vi "Log_Show.vi"() -> (1 "Log Out":string)   [LabVIEW 2020]
panel:
  out "Itterations":i32
  out "ticks":u32
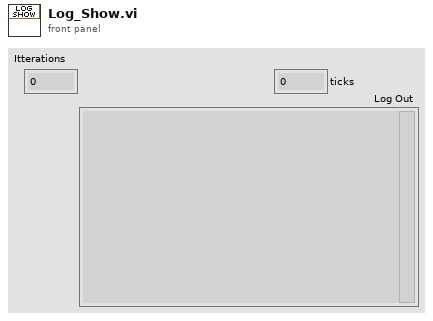
[diagram p1: front panel]
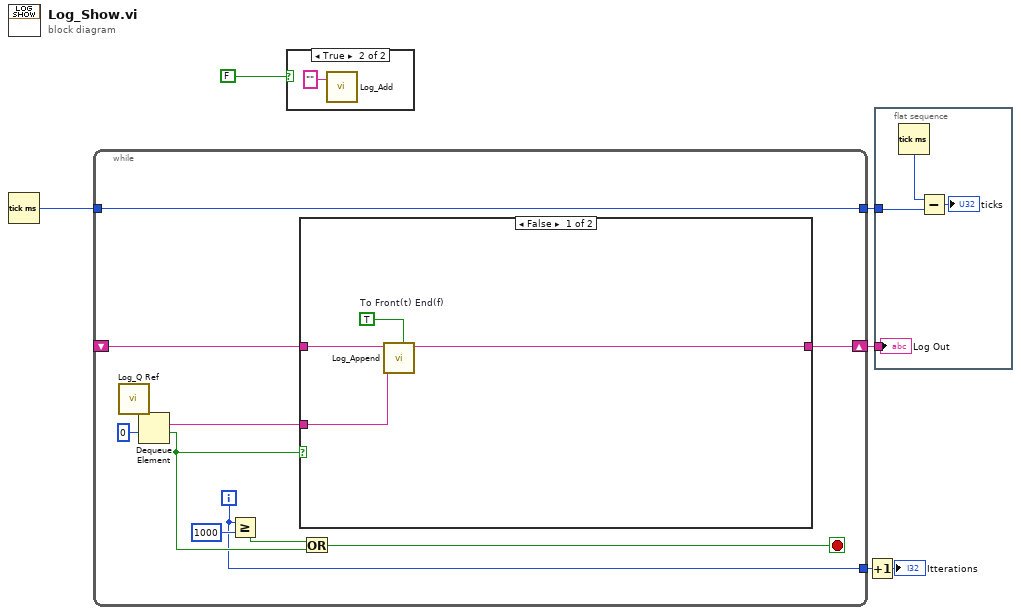
[diagram p0: block diagram]
diagram:
  n1 = Tick Count (ms)() -> (millisecond timer value=w5:u32)
  n2 = while {
    shift-right: [w17] -> w6
    shift-left: _ -> [w15]
    tunnel: w5 -> [w8]
    tunnel: [w8] -> w4
    tunnel: [w7] -> w3
    i -> [w7]
    stop <- w11 stop-if-true
    n3 = call "Log_Q Ref.vi"() -> ("Log Queue"=w16:refnum<queue>)  [unwired: 3 in]
    n4 = Dequeue Element(queue=w16, timeout in ms (-1)=0) -> (element=w14:string, timed out?=w9:bool)  [unwired: 1 in, 2 out]
    n5 = Greater Or Equal?(x=w7, y=1000) -> (x >= y?=w10:bool)
    n6 = case shown="False" w9 {
      tunnel: [w21 w22] -> w17
      tunnel: w15 -> [w20 w22]
      tunnel: w14 -> [w19 _]
      frame False {
        w18 = TRUE  # To Front(t) End(f)
        n7 = call "Log_Append.vi"("To Front(t) End(f)"=w18, "Sting To Append"=w19, "String"=w20) -> ("String Out"=w21:string)  [unwired: 8 in]
      }
      frame True {
      }
    }
    n8 = Or(x=w10, y=w9) -> (x .or. y?=w11:bool)
  }
  n9 = case shown="True" FALSE {
    frame False {
    }
    frame True {
      n10 = call "Log_Add.vi"("Log"="") -> ()  [unwired: 3 in]
    }
  }
  n11 = Increment(x=w3) -> (x+1=→"Itterations":i32)
  n12 = flat-sequence {
    tunnel: w6 -> [w27]
    tunnel: w4 -> [w25]
    frame #0 {
      n13 = Tick Count (ms)() -> (millisecond timer value=w26:u32)
      n14 = Subtract(x=w26, y=w25) -> (x-y=→"ticks":u32)
      "Log Out" <- w27
    }
  }
